vi "is_done.vi"(8 "error in (no error)":errorcluster, 11 "HSDIO in":refnum<class "HSDIO.lvclass">) -> (0 "error out":errorcluster, 2 "HSDIO is done?":bool caption="done", 3 "HSDIO out":refnum<class "HSDIO.lvclass">)   [LabVIEW 2013, in "HSDIO.lvclass"]
uses:
  HSDIO.lvclass
  HSDIO.lvclass/HSDIO.ctl
  Globals.vi
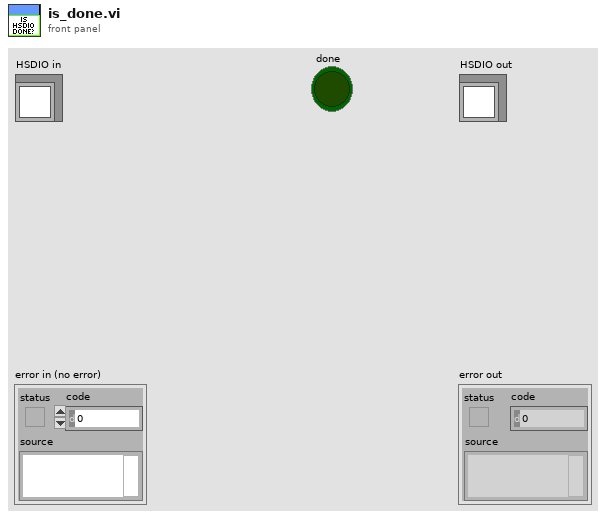
[diagram p1: front panel]
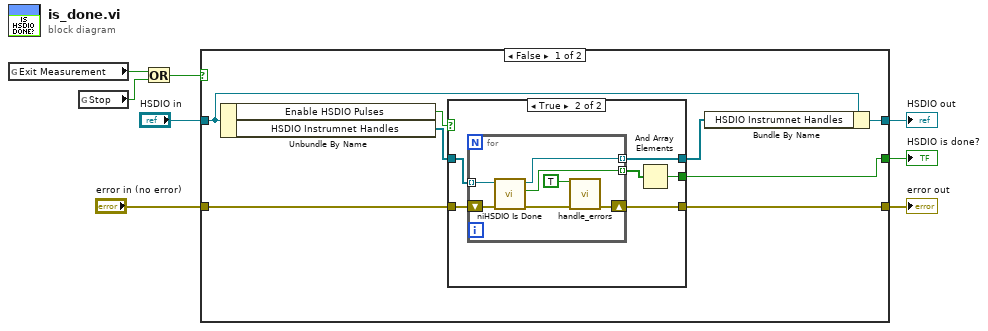
[diagram p0: block diagram]
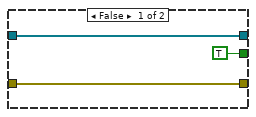
[diagram p2: hidden frame]
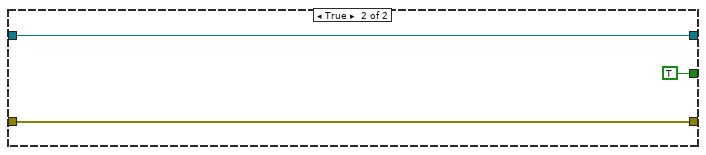
[diagram p3: hidden frame]
diagram:
  n1 = global read "Globals.vi" "Exit Measurement"() -> (w3:bool)
  n2 = global read "Globals.vi" "Stop"() -> (w4:bool)
  n3 = Or(x=w3, y=w4) -> (x .or. y?=w2:bool)
  n4 = case shown="False" w2 {
    tunnel: [w12 w34] -> w8
    tunnel: [w15 w35] -> w6
    tunnel: "HSDIO in" -> [w16 w35]
    tunnel: "error in (no error)" -> [w10 w34]
    tunnel: [w9 TRUE ("done")] -> w1
    frame False {
      n5 = Unbundle By Name(w16) -> ("Enable HSDIO Pulses"=w14:bool, "HSDIO Instrumnet Handles"=w13:refnum<k15>[])
      n6 = case shown="True" w14 {
        tunnel: w13 -> [w19 w25]
        tunnel: w10 -> [w18 w24]
        tunnel: [w18 w22] -> w12
        tunnel: [w19 w23] -> w11
        tunnel: [TRUE ("done") w20] -> w9
        frame False {
        }
        frame True {
          n7 = for {
            tunnel: w25 -> [w32] mode=indexing
            tunnel: [w30] -> w23 mode=indexing
            tunnel: [w29] -> w21 mode=indexing
            shift-right: [w27] -> w22
            shift-left: w24 -> [w31]
            n8 = call <instrlib>:"niHSDIO Is Done.vi"("error in (no error)"=w31, "instrument handle"=w32) -> ("error out"=w28:errorcluster, "done"=w29:bool, "instrument handle out"=w30:refnum<k15>)  [unwired: 7 in]
            n9 = call "handle_errors.vi"("Exit Operation"=TRUE ("Exit Measurement"), "error in (no error)"=w28) -> ("error out"=w27:errorcluster)  [unwired: 13 in]
          }
          n10 = And Array Elements(Boolean array=w21) -> (logical AND=w20:bool)
        }
      }
      n11 = Bundle By Name(cluster=w16, "HSDIO Instrumnet Handles"=w11) -> (w15:refnum<class "HSDIO.lvclass">)
    }
    frame True {
    }
  }
  "error out" <- w8
  "HSDIO out" <- w6
  "HSDIO is done?" <- w1
